vi "MirrorImage.vi"(2 "input":dbl[](array[numeric]) format="%.2f", 3 "neg?":bool) -> (0 "output":dbl[](array[numeric]) format="%.2f")   [LabVIEW 2022 SP3]
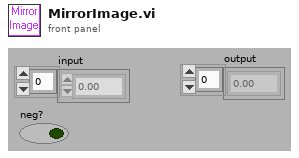
[diagram p1: front panel]
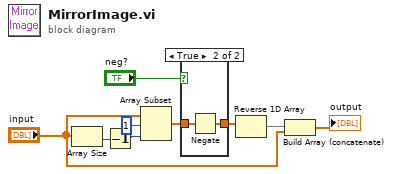
[diagram p0: block diagram]
diagram:
  n1 = Array Size(array="input") -> (size(s)=w2:i32)
  n2 = Decrement(x=w2) -> (x-1=w3:i32)
  n3 = Array Subset(array="input", index=1, length=w3) -> (w5:dbl[])
  n4 = case shown="True" "neg?" {
    tunnel: [w10 w12] -> w9
    tunnel: w5 -> [w10 w11]
    frame False {
    }
    frame True {
      n5 = Negate(x=w11) -> (-x=w12:dbl[])
    }
  }
  n6 = Reverse 1D Array(array=w9) -> (reversed array=w6:dbl[])
  n7 = Build Array (concatenate)(w6, "input") -> (→"output":dbl[])
